vi "fgv_judgement.vi"(7 "cmd":T2, 8 "error in (no error)":errorcluster, 11 "Test Judgement":T1={"전압 63%[mS] Min"=0.0, "전압 98%[mS] Min"=0.0, "전류 37%[mS] Min"=0.0, "접촉저항[mOhm] Min"=800.0, "출력전류 Irms[mA] Min"=5.0, "전압 63%[mS] Max"=0.0, "전압 98%[mS] Max"=0.0, "전류 37%[mS] Max"=0.0, "접촉저항[mOhm] Max"=0.0, "출력전류 Irms[mA] Max"=0.0}) -> (0 "error out":errorcluster, 3 "Test Judgement 2":T1)   [LabVIEW 2019]
uses:
  _ctrl/rw.ctl
  Judge_RC.ctl
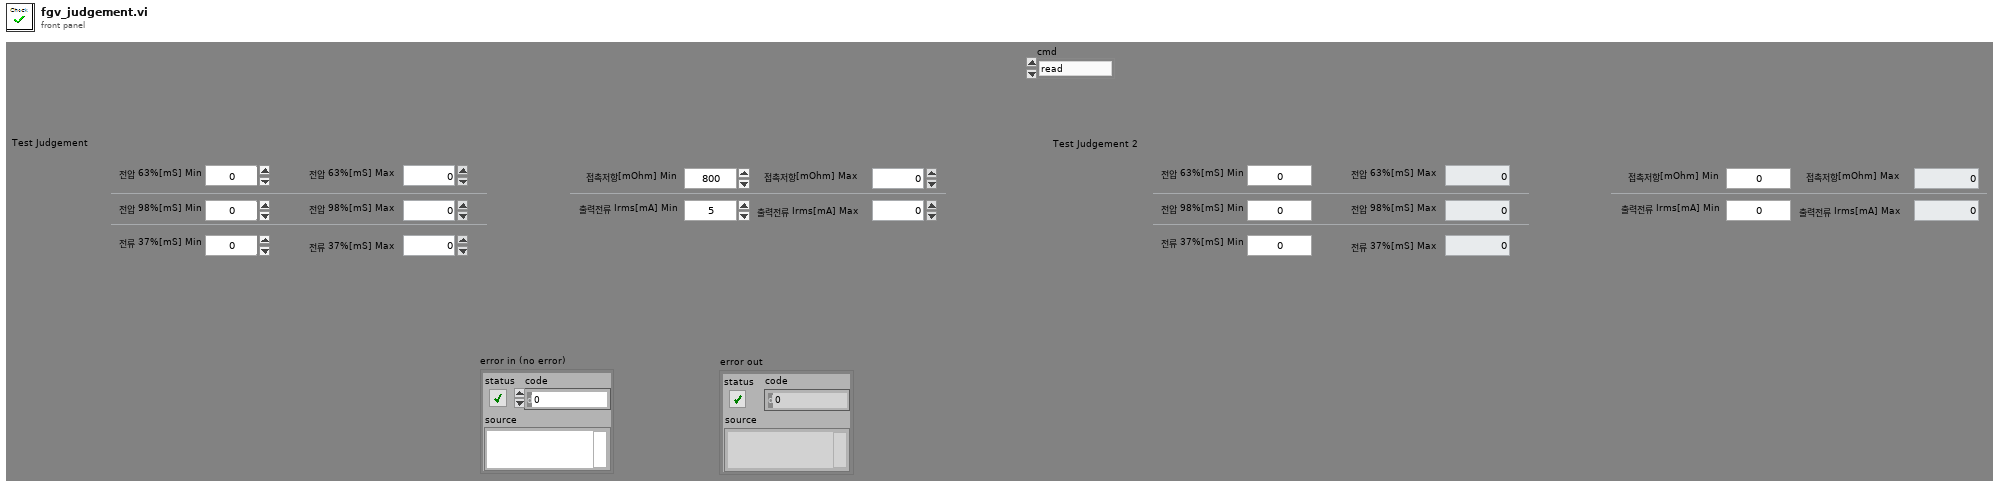
[diagram p1: front panel]
types:
  T1 = typedef "Judge_RC.ctl" = cluster{"전압 63%[mS] Min":dbl, "전압 98%[mS] Min":dbl, "전류 37%[mS] Min":dbl, "접촉저항[mOhm] Min":dbl, "출력전류 Irms[mA] Min":dbl, "전압 63%[mS] Max":dbl, "전압 98%[mS] Max":dbl, "전류 37%[mS] Max":dbl, "접촉저항[mOhm] Max":dbl, "출력전류 Irms[mA] Max":dbl}
  T2 = typedef "rw.ctl" = enum16{"read", "write"}
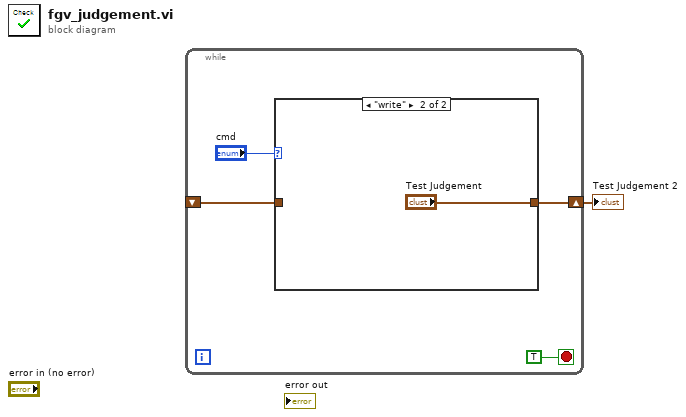
[diagram p0: block diagram]
diagram:
  n1 = while {
    shift-right: [w3] -> w1
    shift-left: _ -> [w2]
    stop <- TRUE stop-if-true
    n2 = case shown="\"write\"" "cmd" {
      tunnel: [w6 "Test Judgement"] -> w3
      tunnel: w2 -> [w6 _]
      frame "read", Default {
      }
      frame "write" {
      }
    }
  }
  "Test Judgement 2" <- w1
